vi "校准测试单次测试.vi"(7 "Limit":dbl, 8 "error in (no error)":errorcluster, 9 "out":i32=1, 11 "in":i32=2) -> (0 "error out":errorcluster)   [LabVIEW 2015]
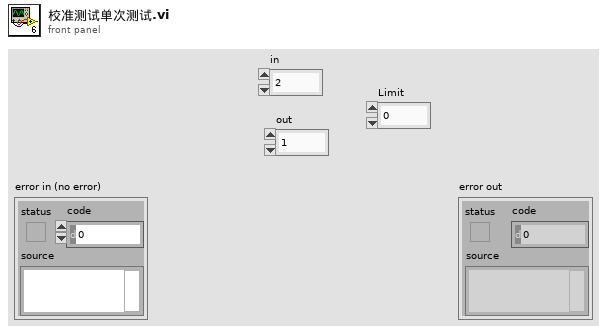
[diagram p1: front panel]
types:
  T1 = typedef "直通基准state.ctl" = enum16{"Idle", "开始消息", "切换开关", "网分测量", "数据库操作", "结束消息"}
  T2 = cluster{"Freq":dbl[], "S11":dbl[], "S12":dbl[], "S21":dbl[], "S22":dbl[]}
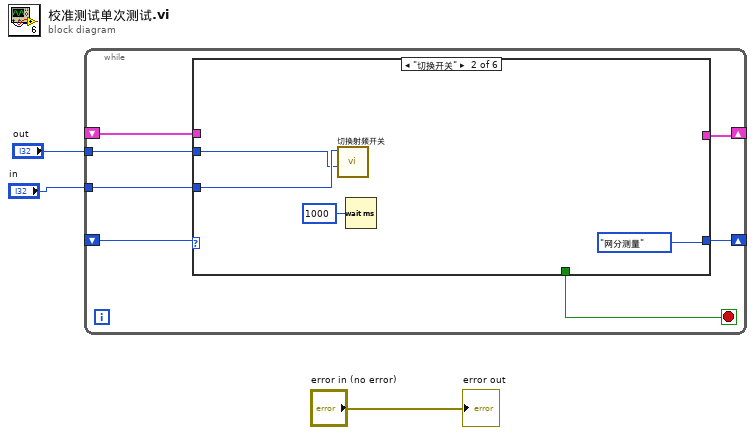
[diagram p0: block diagram]
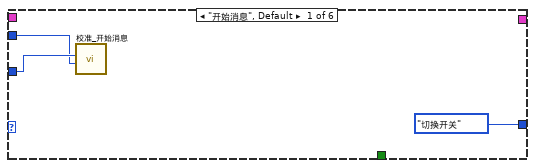
[diagram p2: hidden frame]
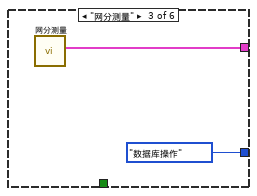
[diagram p3: hidden frame]
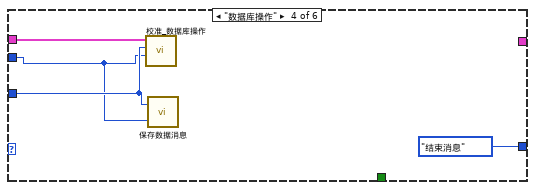
[diagram p4: hidden frame]
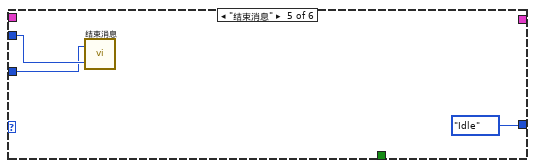
[diagram p5: hidden frame]
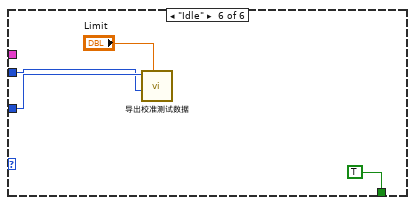
[diagram p6: hidden frame]
diagram:
  n1 = while {
    tunnel: "out" -> [w10]
    tunnel: "in" -> [w9]
    shift-right: [w7] -> _
    shift-left: _ -> [w8]
    shift-right: [w5] -> _
    shift-left: _ -> [w4]
    stop <- w6 stop-if-true
    n2 = case shown="\"切换开关\"" w8 {
      tunnel: w10 -> [w11 w14 _ w20 w25 w28]
      tunnel: w9 -> [w12 w15 _ w21 w24 w29]
      tunnel: [直通基准state."切换开关" ("直通基准State") 直通基准state."网分测量" ("直通基准State") 直通基准state."数据库操作" ("直通基准State") 直通基准state."结束消息" ("直通基准State") 直通基准state."Idle" ("直通基准State") _] -> w7
      tunnel: [_ _ _ _ _ TRUE] -> w6
      tunnel: [_ _ w19 _ _ _] -> w5
      tunnel: w4 -> [_ _ _ w23 _ _]
      frame "开始消息", Default {
        n3 = call "校准_开始消息.vi"("COM"=w11, "A"=w12) -> ()  [unwired: 10 in]
      }
      frame "切换开关" {
        n4 = call "切换射频开关.vi"("COM"=w14, "A"=w15) -> ()  [unwired: 7 in, 3 out]
        n5 = Wait (ms)(milliseconds to wait=u32 1000) -> ()  [unwired: 1 out]
      }
      frame "网分测量" {
        n6 = call "网分测量.vi"() -> ("Freq&S"=w19:T2)  [unwired: 11 in]
      }
      frame "数据库操作" {
        n7 = call "校准_数据库操作.vi"("出口"=w20, "进口"=w21, "Freq&S"=w23) -> ()  [unwired: 8 in, 1 out]
        n8 = call "保存数据消息.vi"("COM"=w20, "A"=w21) -> ()  [unwired: 1 in]
      }
      frame "结束消息" {
        n9 = call "结束消息.vi"("COM"=w25, "A"=w24) -> ()  [unwired: 1 in]
      }
      frame "Idle" {
        n10 = call "导出校准测试数据.vi"("阀值"="Limit", "COM"=w28, "IN"=w29) -> ()  [unwired: 8 in, 1 out]
      }
    }
  }
  "error out" <- "error in (no error)"
